vi "program seq..vi"(6 "IOList":T3, 7 "Cluster data":T6, 8 "DO":T4, 11 "Filepath":path=path "E:/My Project/2018-2019/Under development/Minda Ind. Switch -ID 144-145/Project/data/trail pro -12.txt") -> (0 "Error Out":errorcluster)   [LabVIEW 2015]
uses:
  Control PB/Active.ctl
  Control PB/deactive.ctl
  Control PB/output control.ctl
  Control PB/input control.ctl
  Control PB/timer.ctl
  Control PB/Remove list.ctl
  Control Button/Exit.ctl
  Control PB/Add_s.ctl
  Control PB/Delete_.ctl
  Control Button/Save.ctl
  Control PB/motor.ctl
  Data Acquisition/PCI-USB-DAQ/Digital out put.ctl
  Control PB/Camera.ctl
  Control PB/Barcode.ctl
  Galobal variable_TI.vi
panel:
  in  "Barcode 2":T1
  out "Step List 4":string[](array[string])
  out "Step List 3":string[](array[string])
  in  "Barcode":T1
  in  "Camera":T2
  out "x <= y?":bool
  out "Cancel":bool
  out "Step List 2":string[](array[string])
  out "Pokayoka Result":cluster{"Sensor Name":string, "Boolean":bool}[](array[cluster])
  in  "Feed Back Channel":i32[](listbox)=[0]
  out "Input":bool[](array[boolean])
  out "Feature List (Out) 2":T5(array[cluster])
  out "error out 2":errorcluster
  in  "Control":bool
  out "Station No":string
  out "Model Name":string
  out "Machine Name":string
  in  "Motor":T7
  in  "Feature List":i32(listbox) caption="Steps List"
  in  "Deletefeature list":T8
  in  "Add feature list":T9
  in  "Deactive":T10
  in  "Active":T11
  in  "Program step":i32(listbox)
  in  "Remove Step":T12
  in  "Wait Time":u32=100 caption="Timer(ms)" max=600000 step=1
  in  "Timer":T13
  in  "Save":T14
  in  "stop":T15
  in  "op Add":T16
  in  "Input Add":T17
  out "Step List":string[](array[string])
  out "output cluster":T18
  in  "Analog":bool
  in  "Analog Input":i32[](listbox)=[0]
  in  "Control Channel":i32[](listbox)=[7]
  in  "Steps":T19(array[cluster])
  in  "Program mode":string="Data"
  out "error out":errorcluster
  out "Feature List (Out)":T20(array[cluster])
  # "Program Sequence Window"
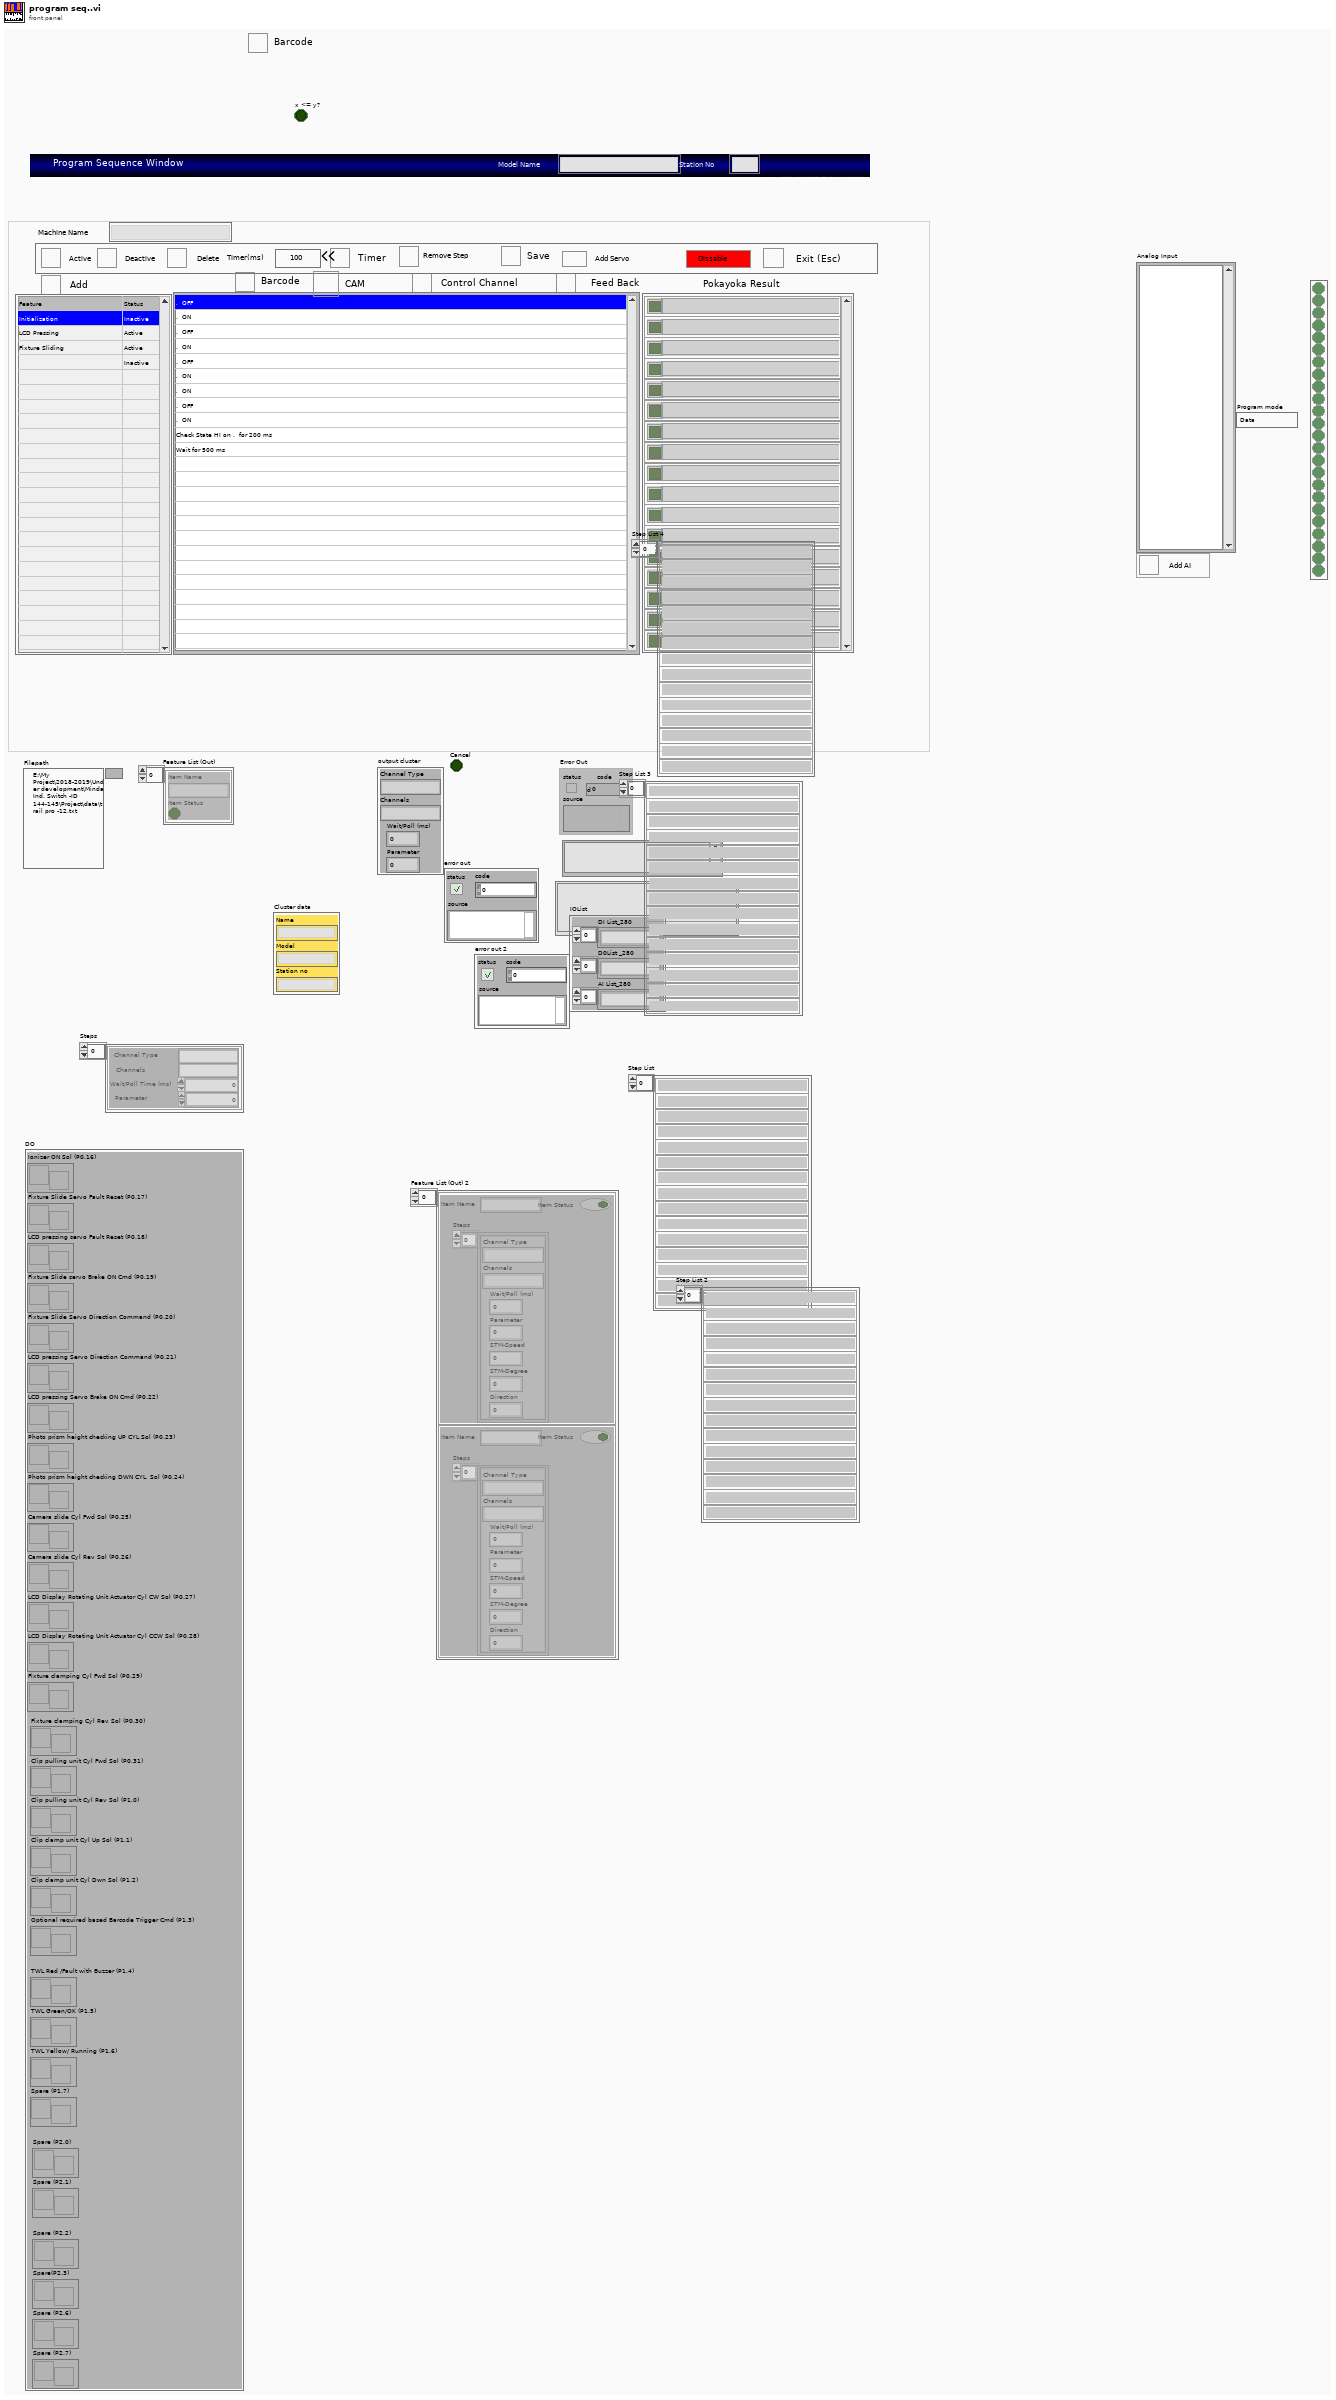
[diagram p1: front panel]
types:
  T1 = typedef "Barcode.ctl" = bool
  T2 = typedef "Camera.ctl" = bool
  T3 = cluster{"DI List_280":string[], "D0List _280":string[], "AI List_280":string[]}
  T4 = typedef "Digital out put.ctl" = cluster{"Ionizer ON Sol (P0.16)":refnum<notifier>, "Fixture Slide Servo Fault Reset (P0.17)":refnum<notifier>, "LCD pressing servo Fault Reset (P0.18)":refnum<notifier>, "Fixture Slide servo Brake ON Cmd (P0.19)":refnum<notifier>, "Fixture Slide Servo Direction Command (P0.20)":refnum<notifier>, "LCD pressing Servo Direction Command (P0.21)":refnum<notifier>, "LCD pressing Servo Brake ON Cmd (P0.22)":refnum<notifier>, "Photo prism height checking UP CYL Sol (P0.23)":refnum<notifier>, "Photo prism height checking DWN CYL  Sol (P0.24)":refnum<notifier>, "Camera slide Cyl Fwd Sol (P0.25)":refnum<notifier>, "Camera slide Cyl Rev Sol (P0.26)":refnum<notifier>, "LCD Display Rotating Unit Actuator Cyl CW Sol (P0.27)":refnum<notifier>, "LCD Display Rotating Unit Actuator Cyl CCW Sol (P0.28)":refnum<notifier>, "Fixture clamping Cyl Fwd Sol (P0.29)":refnum<notifier>, "Fixture clamping Cyl Rev Sol (P0.30)":refnum<notifier>, "Clip pulling unit Cyl Fwd Sol (P0.31)":refnum<notifier>, "Clip pulling unit Cyl Rev Sol (P1.0)":refnum<notifier>, "Clip clamp unit Cyl Up Sol (P1.1)":refnum<notifier>, "Clip clamp unit Cyl Dwn Sol (P1.2)":refnum<notifier>, "Optional required based Barcode Trigger Cmd (P1.3)":refnum<notifier>, "TWL Red /Fault with Buzzer (P1.4)":refnum<notifier>, "TWL Green/OK (P1.5)":refnum<notifier>, "TWL Yellow/ Running (P1.6)":refnum<notifier>, "Spare (P1.7)":refnum<notifier>, "Spare (P2.0)":refnum<notifier>, "Spare (P2.1)":refnum<notifier>, "Spare (P2.2)":refnum<notifier>, "Spare(P2.3)":refnum<notifier>, "Spare (P2.6)":refnum<notifier>, "Spare (P2.7) ":refnum<notifier>}
  T5 = cluster{"Item Name":string, "Item Status":bool, "Steps":cluster{"Channel Type":string, "Channels":string, "Wait/Poll (ms)":u32, "Parameter":u8, "STM-Speed":i32, "STM-Degree":u32, "Direction":u8}[]}[]
  T6 = cluster{"Name":string, "Model":string, "Station no":string}
  T7 = typedef "motor.ctl" = bool
  T8 = typedef "Delete_.ctl" = bool
  T9 = typedef "Add_s.ctl" = bool
  T10 = typedef "deactive.ctl" = bool
  T11 = typedef "Active.ctl" = bool
  T12 = typedef "Remove list.ctl" = bool
  T13 = typedef "timer.ctl" = bool
  T14 = typedef "Save.ctl" = bool
  T15 = typedef "Exit.ctl" = bool
  T16 = typedef "output control.ctl" = bool
  T17 = typedef "input control.ctl" = bool
  T18 = cluster{"Channel Type":string, "Channels":string, "Wait/Poll (ms)":u32, "Parameter":u8}
  T19 = cluster{"Channel Type":string, "Channels":string, "Wait/Poll Time (ms)":u32, "Parameter":u8}[]
  T20 = cluster{"Item Name":string, "Item Status":bool}[]
  T21 = cluster{"Channel Type":string, "Channels":string, "Wait/Poll (ms)":u32, "Parameter":u8, "STM-Speed":i32, "STM-Degree":i32, "Direction":u8}
  T22 = cluster{"Item Name":string, "Item Status":bool, "Steps":cluster{"Channel Type":string, "Channels":string, "Wait/Poll (ms)":u32, "Parameter":u8, "STM-Speed":i32, "STM-Degree":u32, "Direction":u8}[]}
  T23 = cluster{"Channel Type":string, "Channels":string, "Wait/Poll (ms)":u32, "Parameter":u8, "STM-Speed":i32, "STM-Degree":u32, "Direction":u8}[]
  T24 = cluster{"Item Name":string, "Active":T11, "Steps":cluster{"Channel Type":string, "Channels":string, "Wait/Poll (ms)":u32, "Parameter":u8, "STM-Speed":i32, "STM-Degree":u32, "Direction":u8}[]}
  T25 = cluster{"Channel Type":string, "Channels":string, "Wait/Poll (ms)":u32, "Parameter":u8, "STM-Speed":i32, "STM-Degree":i32, "Direction":u8}[]
  T26 = cluster{"Feature name ":string, bool, cluster{"Channel Type":string, "Channels":string, "Wait/Poll (ms)":u32, "Parameter":u8, "STM-Speed":i32, "STM-Degree":i32, "Direction":u8}[]}
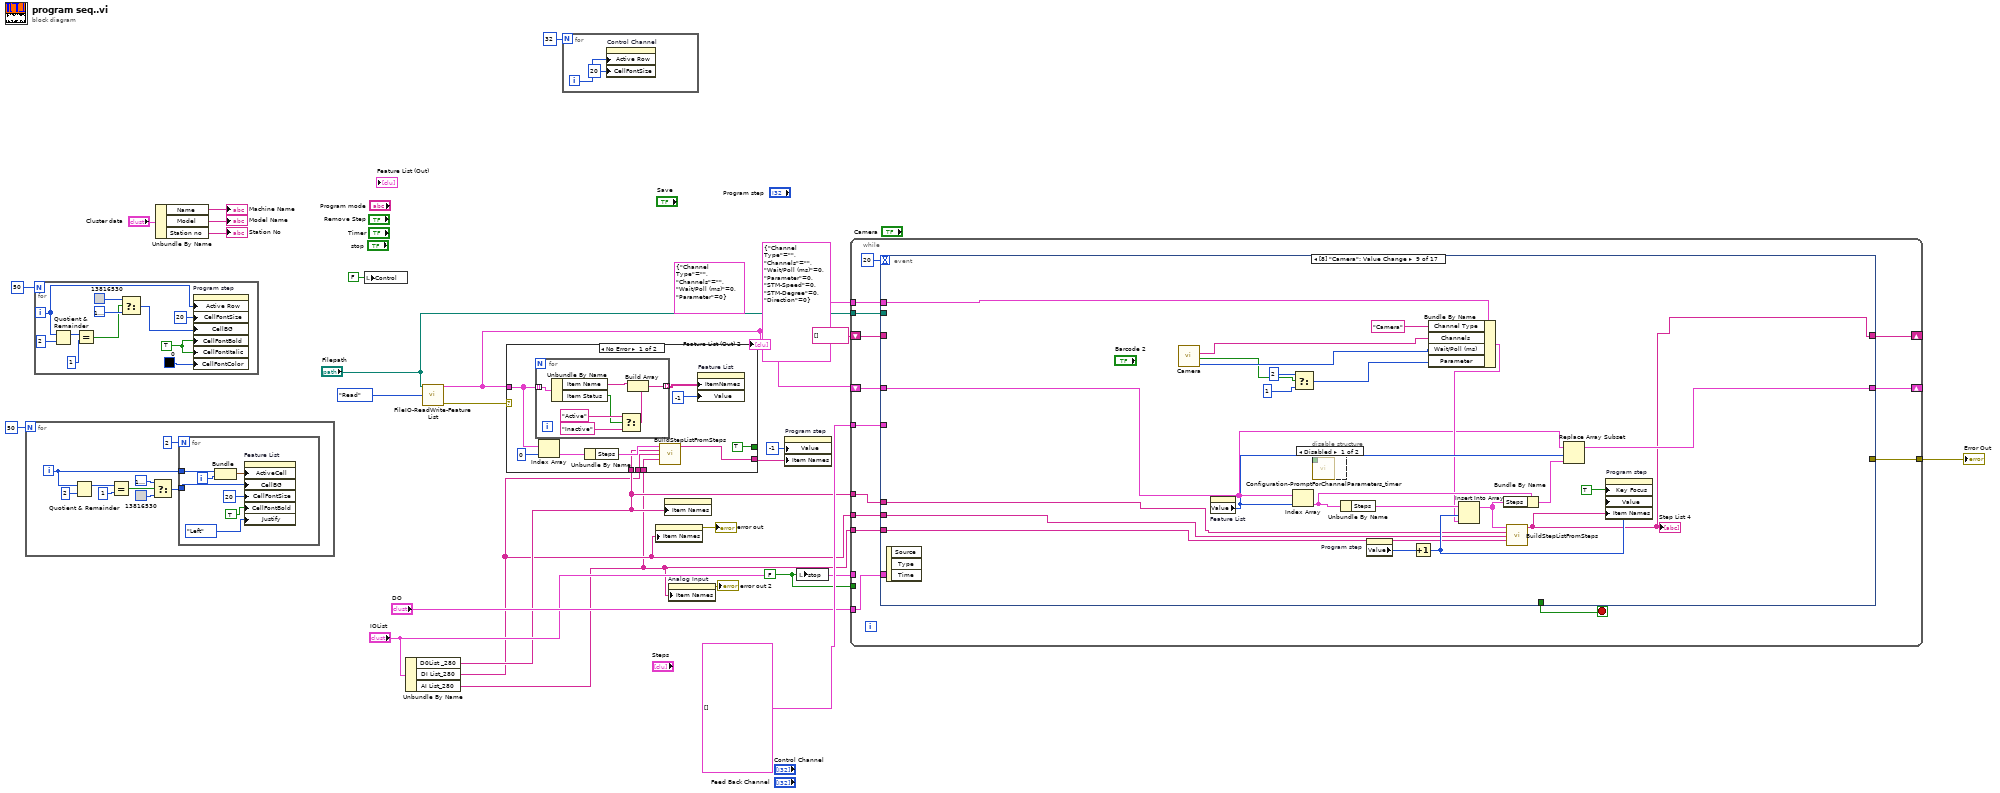
[diagram p0: block diagram]
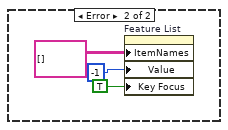
[diagram p2: hidden frame]
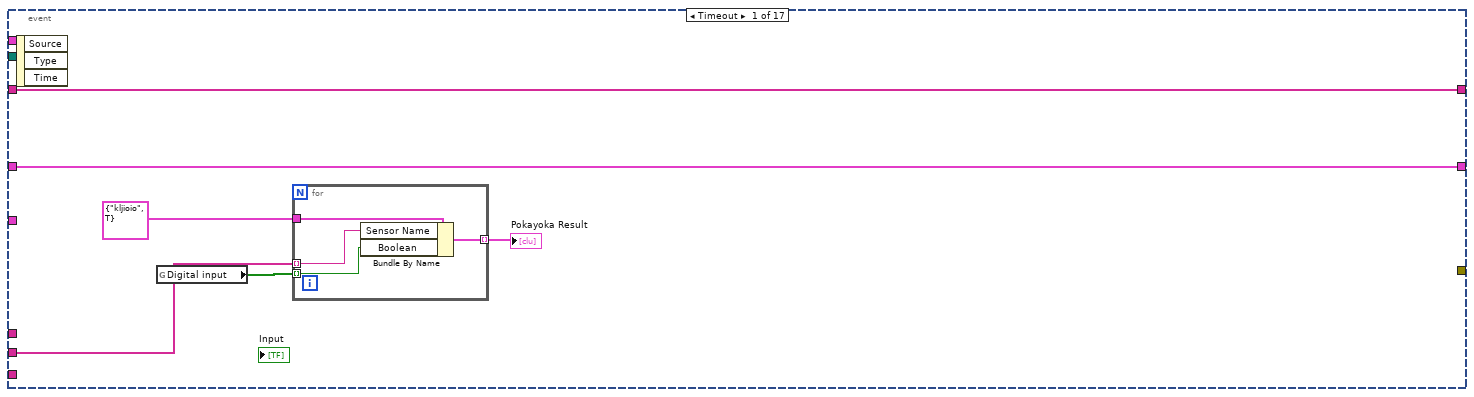
[diagram p3: hidden frame]
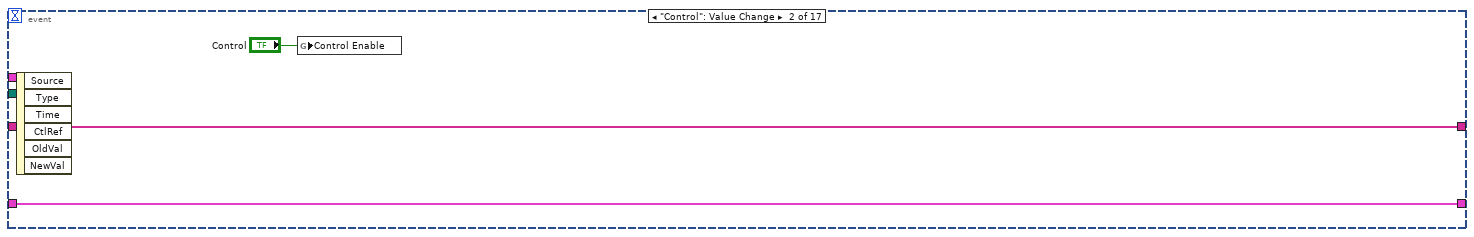
[diagram p4: hidden frame]
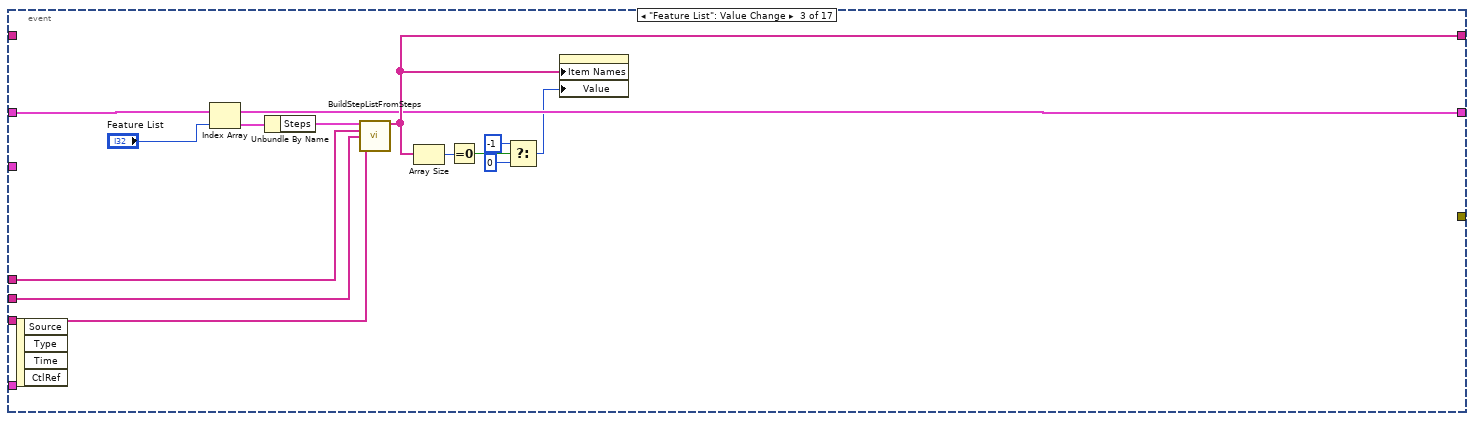
[diagram p5: hidden frame]
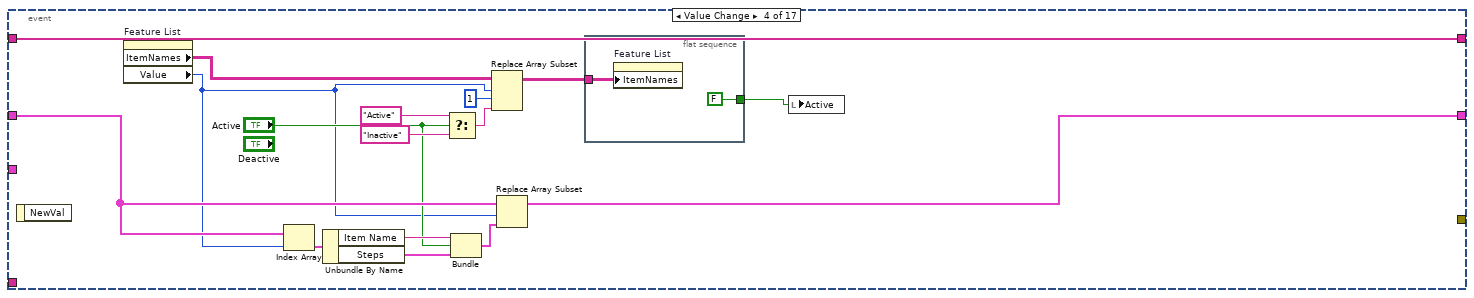
[diagram p6: hidden frame]
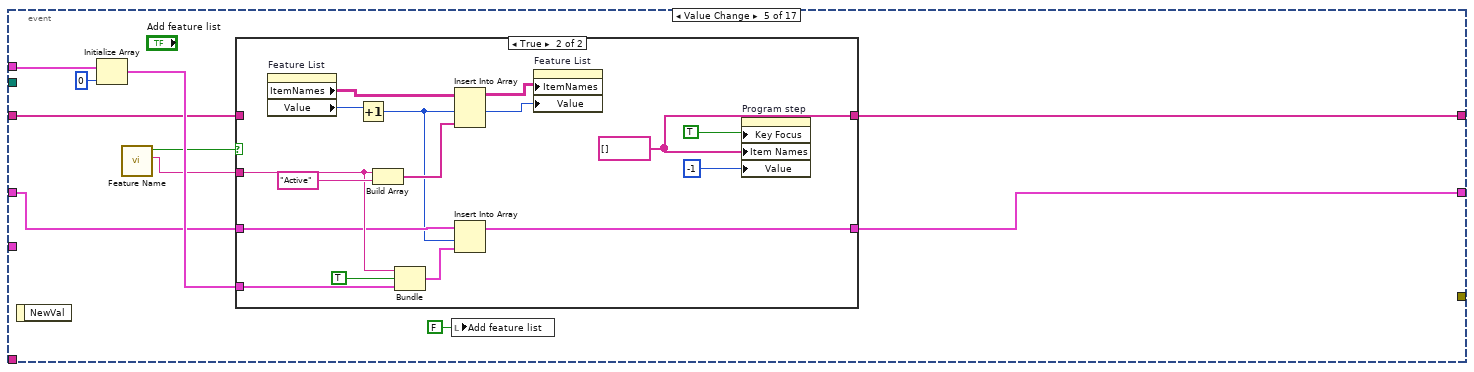
[diagram p7: hidden frame]
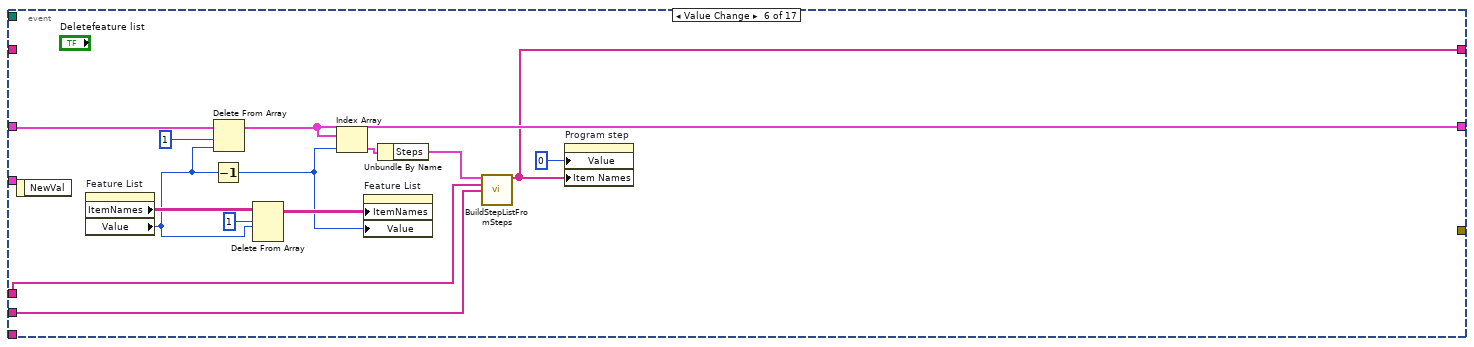
[diagram p9: hidden frame]
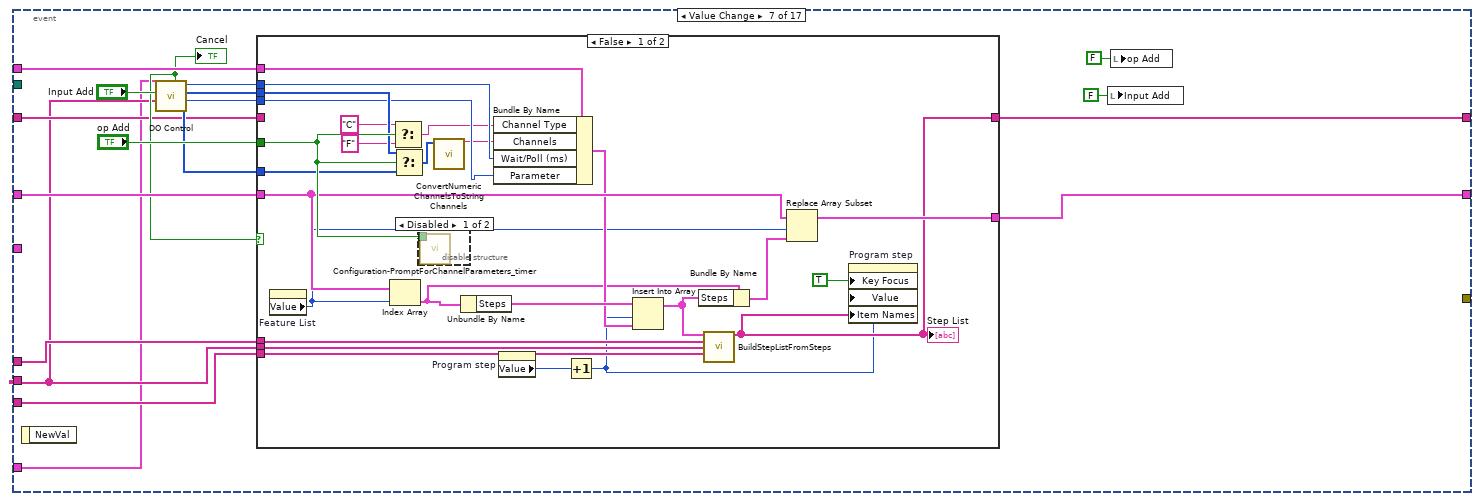
[diagram p10: hidden frame]
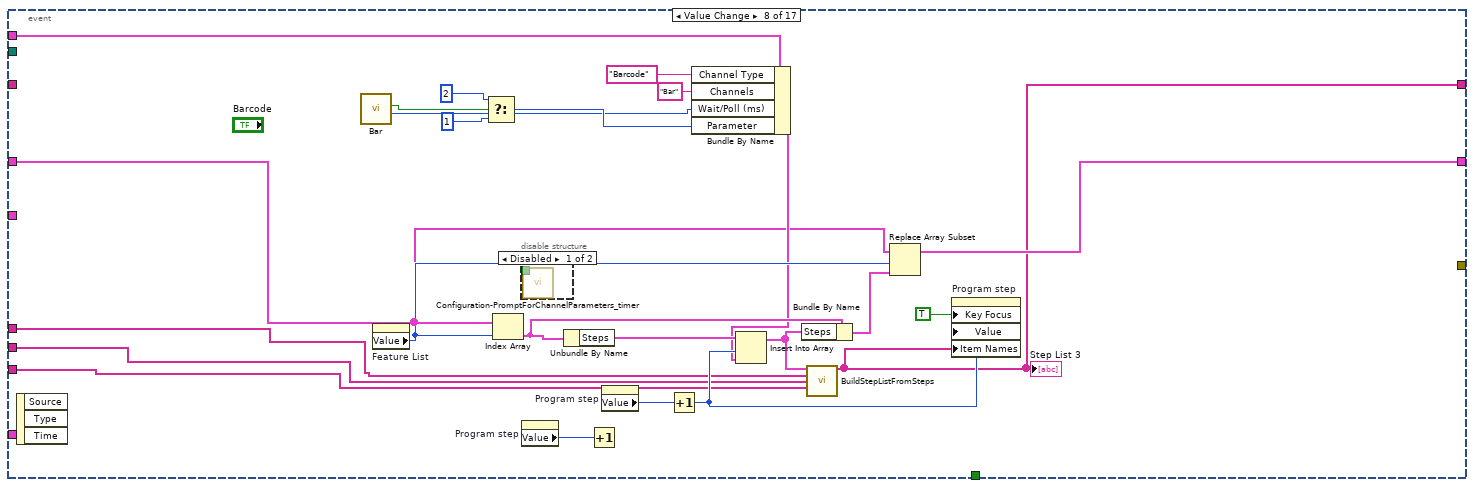
[diagram p13: hidden frame]
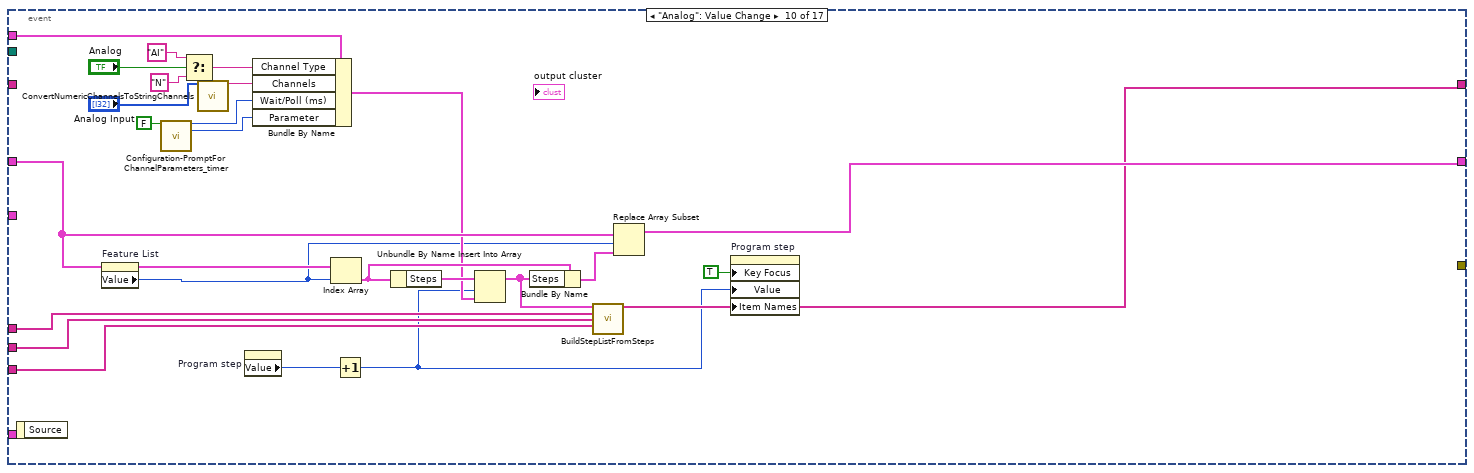
[diagram p16: hidden frame]
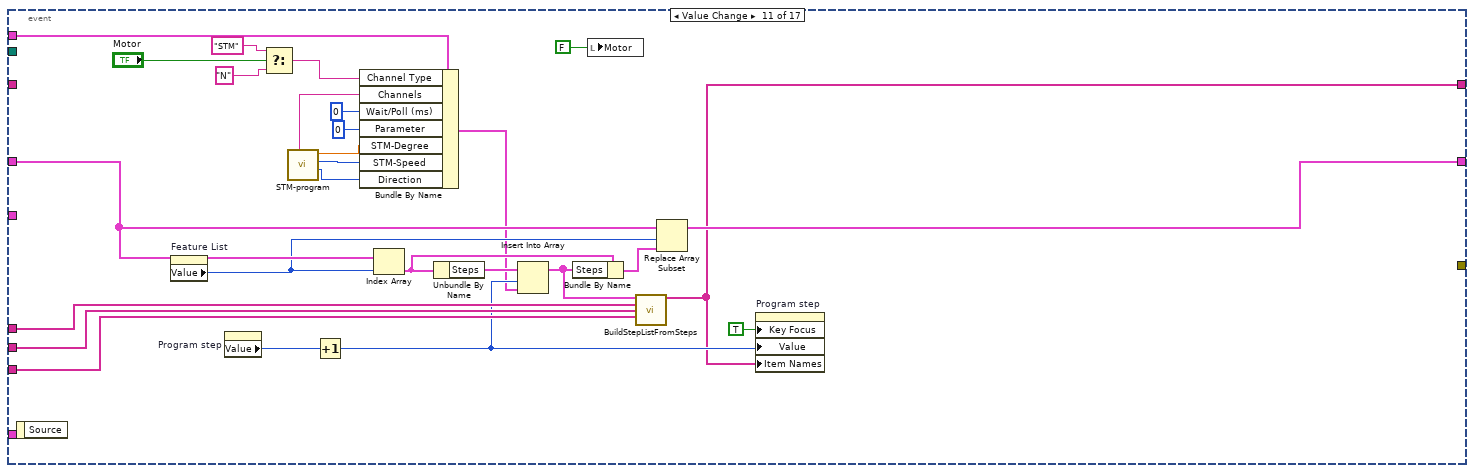
[diagram p17: hidden frame]
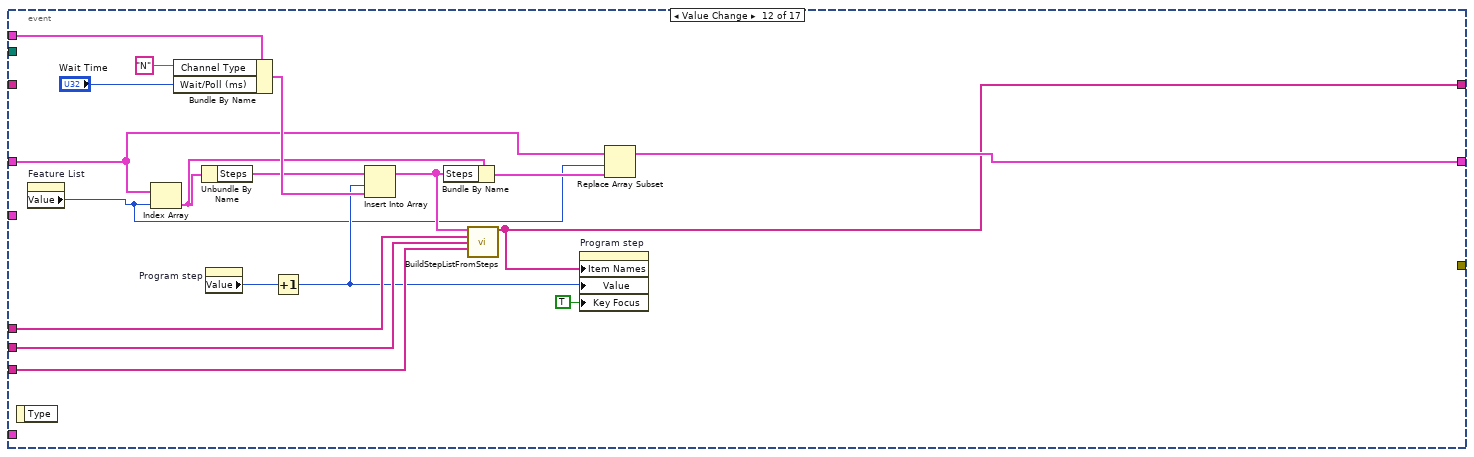
[diagram p18: hidden frame]
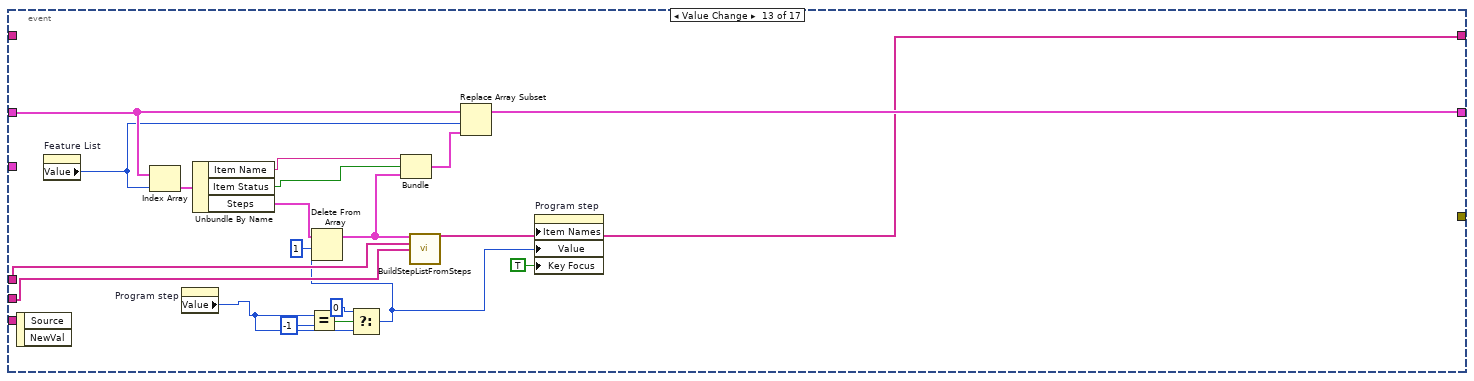
[diagram p19: hidden frame]
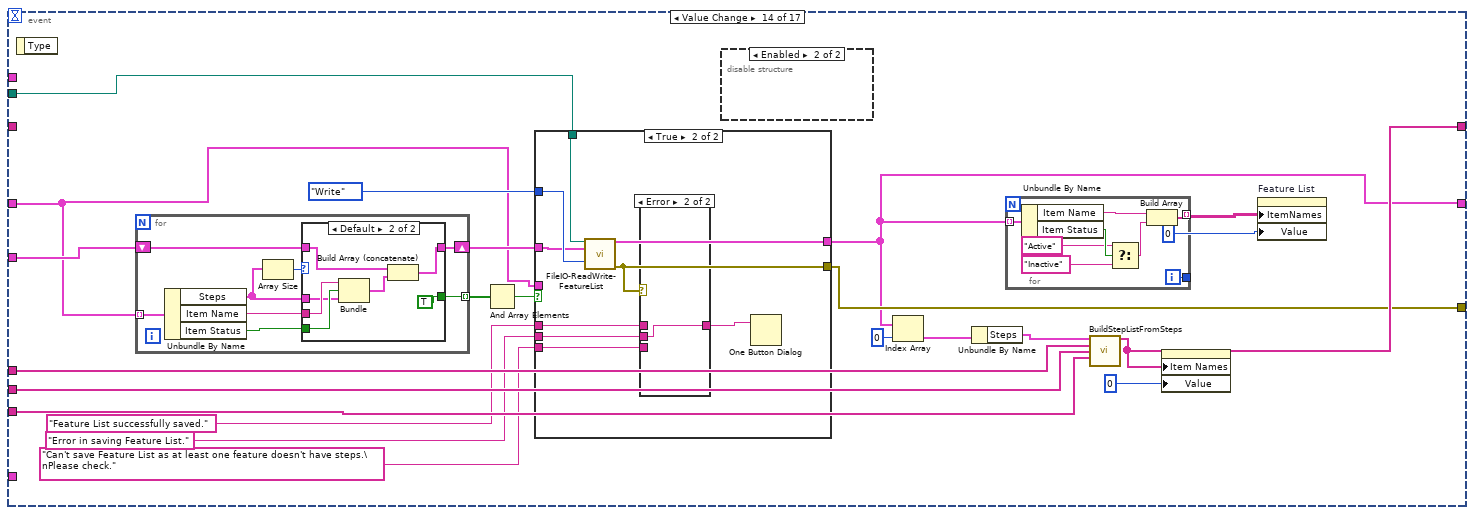
[diagram p20: hidden frame]
diagram:
  w9 = FALSE ("stop")
  (unwired) T18 {"Channel Type"="", "Channels"="", "Wait/Poll (ms)"=0, "Parameter"=0} ("Step")
  n1 = for {
    N: 50 -> [_]
    i -> [w34]
    n2 = Quotient & Remainder(x=w34, y=2) -> (x-y*floor(x/y)=w32:i32)  [unwired: 1 out]
    n3 = Equal?(x=w32, y=1) -> (x = y?=w30:bool)
    n4 = Select(t=u32 16777225 ("Color Box"), s=w30, f=u32 13816530 ("Color Box")) -> (s? t:f=w27:u32)
    n5 = for {
      N: 2 -> [_]
      tunnel: w34 -> [w42]
      tunnel: w27 -> [w39]
      i -> [w41]
      n6 = Bundle(w42, w41) -> (w40:cluster{i32, i32})  [unwired: 1 in]
      n7 = property on="Feature List" class="MCListbox (strict)"("ActiveCell"=w40, "CellBG"=w39, "CellFontSize"=u32 20 ("Active Cell:Cell Font:Size"), "CellFontBold"=TRUE ("Active Cell:Cell Font:Bold"), "Justify"=enum16{"Left", "Center", "Right"}."Left" ("Active Cell:Cell Justification")) -> ()  [unwired: 2 in, 2 out]
    }
  }
  n8 = for {
    N: 50 -> [_]
    i -> [w47]
    w44 = TRUE
    n9 = Quotient & Remainder(x=w47, y=2) -> (x-y*floor(x/y)=w50:i32)  [unwired: 1 out]
    n10 = Equal?(x=w50, y=1) -> (x = y?=w48:bool)
    n11 = Select(t=u32 13816530 ("Color Box"), s=w48, f=u32 16777226 ("Color Box")) -> (s? t:f=w45:u32)
    n12 = property on="Program step" class="LstBox (strict)"("Active Row"=w47, "CellFontSize"=u32 20 ("Active Row:Cell Font:Size"), "CellBG"=w45, "CellFontBold"=w44, "CellFontItalic"=w44, "CellFontColor"=u32 0 ("Color Box")) -> ()  [unwired: 2 in, 2 out]
  }
  n13 = Unbundle By Name("Cluster data") -> ("Name"=→"Machine Name":string, "Model"=→"Model Name":string, "Station no"=→"Station No":string)
  n14 = local write "Control"(FALSE ("Control")) -> ()
  n15 = Unbundle By Name("IOList") -> ("D0List _280"=w4:string[], "DI List_280"=w3:string[], "AI List_280"=w2:string[])
  n16 = call "FileIO-ReadWrite-FeatureList.vi"("Filepath"="Filepath", "Read/Write"=enum16{"Read", "Write"}."Read") -> ("Feature List (Out)"=w17:T5, "Error Out"=w21:errorcluster)  [unwired: 12 in]
  "Feature List (Out) 2" <- w17
  n17 = case shown="No Error" w21 {
    tunnel: w17 -> [w64 _]
    tunnel: w4 -> [w60 _]
    tunnel: w3 -> [w59 _]
    tunnel: w2 -> [w58 _]
    tunnel: [w57 _] -> w20
    tunnel: [TRUE ("Key Focus") _] -> _
    frame No Error {
      n18 = for {
        tunnel: w64 -> [w71] mode=indexing
        tunnel: [w65] -> w55 mode=indexing
        n19 = Unbundle By Name(w71) -> ("Item Name"=w67:string, "Item Status"=w68:bool)
        n20 = Select(t="Active", s=w68, f="Inactive") -> (s? t:f=w66:string)
        n21 = Build Array(w67, w66) -> (w65:string[])
      }
      n22 = Index Array(array=w64, index=0) -> (element=w62:T22)
      n23 = Unbundle By Name(w62) -> ("Steps"=w61:T23)
      n24 = call "BuildStepListFromSteps.vi"("Steps"=w61, "Control Channels"=w60, "Feedback Channels"=w59, "AI"=w58) -> ("Step List"=w57:string[])  [unwired: 11 in]
      n25 = property on="Feature List" class="MCListbox (strict)"("ItemNames"=w55, "Value"=-1 ("Feautre list")) -> ()  [unwired: 2 in, 2 out]
    }
    frame Error {
      n26 = property on="Feature List" class="MCListbox (strict)"("ItemNames"=string[][] [] ("Item Names"), "Value"=-1 ("Feautre list"), "Key Focus"=TRUE) -> ()  [unwired: 2 in, 2 out]
    }
  }
  n27 = for {
    N: 32 -> [_]
    i -> [w76]
    n28 = property on="Control Channel" class="LstBox (strict)"("Active Row"=w76, "CellFontSize"=u32 20 ("Active Row:Cell Font:Size")) -> ()  [unwired: 2 in, 2 out]
  }
  n29 = property on="Feed Back Channel" class="LstBox (strict)"("Item Names"=w3) -> (error out=→"error out":errorcluster)  [unwired: 2 in, 1 out]
  n30 = property on="Control Channel" class="LstBox (strict)"("Item Names"=w4) -> ()  [unwired: 2 in, 2 out]
  n31 = property on="Analog Input" class="LstBox (strict)"("Item Names"=w2) -> (error out=→"error out 2":errorcluster)  [unwired: 2 in, 1 out]
  n32 = property on="Program step" class="LstBox (strict)"("Value"=-1 ("Step feautre list"), "Item Names"=w20) -> ()  [unwired: 2 in, 2 out]
  n33 = local write "stop"(w9) -> ()
  n34 = while {
    shift-right: [w88] -> _
    shift-left: w17 -> [w79]
    tunnel: T21 {"Channel Type"="", "Channels"="", "Wait/Poll (ms)"=0, "Parameter"=0, "STM-Speed"=0, "STM-Degree"=0, "Direction"=0} ("Step") -> [w89]
    shift-right: [w87] -> _
    shift-left: string[] [] ("Step List") -> [w86]
    tunnel: w4 -> [w85]
    tunnel: w3 -> [w84]
    tunnel: [w83] -> w24
    tunnel: w2 -> [w82]
    tunnel: T5 [] ("Feature List (Out) 2") -> [w81]
    tunnel: "Filepath" -> [w80]
    tunnel: w9 -> [_]
    tunnel: "DO" -> [w78]
    tunnel: "IOList" -> [_]
    stop <- w90 stop-if-true
    n35 = event shown="[8] \"Camera\": Value Change" {
      selector: _ -> [_ _ _ _ _ _ _ _ _ _ _ _ _ _ _ _ _]
      dyn-events: _ -> [_ _ _ _ _ _ _ _ _ _ _ _ _ _ _ _ _]
      timeout: 20 -> [_ _ _ _ _ _ _ _ _ _ _ _ _ _ _ _ _]
      tunnel: [_ _ _ _ _ _ _ _ _ _ _ _ _ _ TRUE ("stop") _ TRUE ("Discard?")] -> w90
      tunnel: w79 -> [w96 w102 w107 w124 w141 w173 w190 w226 w253 w281 w311 w332 w354 w363 w423 w445 w522]
      tunnel: w89 -> [_ _ _ _ w144 _ w193 w246 w257 w288 w316 w341 _ _ _ w446 _]
      tunnel: [w96 w102 w107 w122 w140 w172 w191 w225 w252 w276 w303 w331 w353 w365 w423 w441 w522] -> w88
      tunnel: [w95 w103 w110 w121 w137 w167 w188 w224 w251 w275 w302 w328 w348 w380 w422 w440 w523] -> w87
      tunnel: w86 -> [w95 w103 _ w121 w136 _ w178 _ _ _ _ _ _ _ w422 w439 w523]
      tunnel: w85 -> [_ _ w109 _ _ w169 w189 w227 w254 w278 w308 w330 w350 w382 _ w442 _]
      tunnel: w84 -> [w94 _ w108 _ _ w168 w177 w228 w255 w279 w307 w329 w349 w381 _ w443 _]
      tunnel: [_ _ _ _ _ _ _ _ _ _ _ _ _ w373 _ _ _] -> w83
      tunnel: w82 -> [_ _ w106 _ _ _ w187 w229 w256 w280 w306 w327 _ w374 _ w444 _]
      tunnel: w81 -> [_ _ _ _ _ _ _ _ _ _ _ _ _ w379 _ _ _]
      tunnel: w80 -> [_ _ _ _ _ _ _ _ _ _ _ _ _ w364 _ _ _]
      tunnel: w78 -> [_ _ _ _ _ _ w176 _ _ _ _ _ _ _ _ _ _]
      event Timeout {
        n36 = event-data() -> ()  [unwired: 1 in, 3 out]
        n37 = global read "Galobal variable_TI.vi" "Digital input"() -> (w91:bool[])
        n38 = for {
          tunnel: w94 -> [w99] mode=indexing
          tunnel: cluster{"Sensor Name":string, "Boolean":bool} {"Sensor Name"="kljioio", "Boolean"=TRUE} ("Cluster") -> [w100]
          tunnel: [w98] -> w92 mode=indexing
          tunnel: w91 -> [w97] mode=indexing
          n39 = Bundle By Name(cluster=w100, "Sensor Name"=w99, "Boolean"=w97) -> (w98:cluster{"Sensor Name":string, "Boolean":bool})
        }
        "Pokayoka Result" <- w92
      }
      event "Control": Value Change {
        n40 = event-data() -> ()  [unwired: 1 in, 6 out]
        n41 = global write "Galobal variable_TI.vi" "Control Enable"("Control") -> ()
      }
      event "Feature List": Value Change {
        n42 = event-data() -> ()  [unwired: 1 in, 4 out]
        n43 = Index Array(array=w107, index="Feature List") -> (element=w116:T22)
        n44 = Unbundle By Name(w116) -> ("Steps"=w115:T23)
        n45 = call "BuildStepListFromSteps.vi"("Steps"=w115, "Control Channels"=w109, "Feedback Channels"=w108, "AI"=w106) -> ("Step List"=w110:string[])  [unwired: 11 in]
        n46 = Array Size(array=w110) -> (size(s)=w112:i32)
        n47 = Equal To 0?(x=w112) -> (x = 0?=w114:bool)
        n48 = Select(t=-1 ("Step List"), s=w114, f=0 ("Step List")) -> (s? t:f=w105:i32)
        n49 = property on="Program step" class="LstBox (strict)"("Item Names"=w110, "Value"=w105) -> ()  [unwired: 2 in, 2 out]
      }
      event Value Change {
        n50 = event-data() -> ()  [unwired: 1 in, 1 out]
        n51 = property on="Feature List" class="MCListbox (strict)"() -> ("ItemNames"=w120:string[][], "Value"=w118:i32)  [unwired: 2 in, 2 out]
        n52 = Index Array(array=w124, index=w118) -> (element=w130:T22)
        n53 = Unbundle By Name(w130) -> ("Item Name"=w131:string, "Steps"=w132:T23)
        n54 = Select(t="Active", s="Active", f="Inactive" ("element")) -> (s? t:f=w127:string)
        n55 = Bundle("Item Name"=w131, "Active"="Active", "Steps"=w132) -> (w129:T24)  [unwired: 1 in]
        n56 = Replace Array Subset(array=w120, new element=w127, index (row)=w118, index (col)=1 ("disabled index (col)")) -> (w119:string[][])
        n57 = Replace Array Subset(array=w124, new element=w129, index=w118) -> (w122:T5)
        n58 = flat-sequence {
          tunnel: w119 -> [w134]
          tunnel: [T11 FALSE ("Active")] -> w117
          frame #0 {
            n59 = property on="Feature List" class="MCListbox (strict)"("ItemNames"=w134) -> ()  [unwired: 2 in, 2 out]
          }
        }
        n60 = local write "Active"(w117) -> ()
      }
      event Value Change {
        n61 = event-data() -> ()  [unwired: 1 in, 1 out]
        n62 = Initialize Array(w144, 0 ("dimension size")) -> (w142:T25)
        n63 = call "Feature Name.vi"() -> ("Feature name"=w138:string, "Out"=w139:bool)  [unwired: 10 in]
        n64 = case shown="True" w139 {
          tunnel: w142 -> [_ w160]
          tunnel: w141 -> [w146 w155]
          tunnel: [w146 w157] -> w140
          tunnel: w138 -> [_ w156]
          tunnel: [w145 w153] -> w137
          tunnel: w136 -> [w145 _]
          frame False {
          }
          frame True {
            w153 = string[] [] ("Item Names")
            n65 = property on="Feature List" class="MCListbox (strict)"() -> ("ItemNames"=w150:string[][], "Value"=w147:i32)  [unwired: 2 in, 2 out]
            n66 = Increment(x=w147) -> (x+1=w148:i32)
            n67 = Build Array(w156, "Active") -> (w151:string[])
            n68 = Bundle("Feature name"=w156, TRUE, w160) -> (w158:T26)  [unwired: 1 in]
            n69 = Insert Into Array(array=w150, index (row)=w148, new element=w151) -> (w149:string[][])  [unwired: 1 in]
            n70 = Insert Into Array(array=w155, index=w148, new element=w158) -> (w157:T5)
            n71 = property on="Feature List" class="MCListbox (strict)"("ItemNames"=w149, "Value"=w148) -> ()  [unwired: 2 in, 2 out]
            n72 = property on="Program step" class="LstBox (strict)"("Key Focus"=TRUE, "Item Names"=w153, "Value"=-1 ("Step feautre list")) -> ()  [unwired: 2 in, 2 out]
          }
        }
        n73 = local write "Add feature list"(FALSE ("Add feature list")) -> ()
      }
      event Value Change {
        n74 = event-data() -> ()  [unwired: 1 in, 1 out]
        n75 = property on="Feature List" class="MCListbox (strict)"() -> ("ItemNames"=w165:string[][], "Value"=w164:i32)  [unwired: 2 in, 2 out]
        n76 = Decrement(x=w164) -> (x-1=w162:i32)
        n77 = Delete From Array(array=w173, length=1, index=w164) -> (array with subset deleted=w172:T5)  [unwired: 1 out]
        n78 = Delete From Array(array=w165, length=1, index (row)=w164) -> (array with subset deleted=w163:string[][])  [unwired: 1 in, 1 out]
        n79 = Index Array(array=w172, index=w162) -> (element=w171:T22)
        n80 = property on="Feature List" class="MCListbox (strict)"("ItemNames"=w163, "Value"=w162) -> ()  [unwired: 2 in, 2 out]
        n81 = Unbundle By Name(w171) -> ("Steps"=w170:T23)
        n82 = call "BuildStepListFromSteps.vi"("Steps"=w170, "Control Channels"=w169, "Feedback Channels"=w168) -> ("Step List"=w167:string[])  [unwired: 12 in]
        n83 = property on="Program step" class="LstBox (strict)"("Value"=0 ("Step feautre list"), "Item Names"=w167) -> ()  [unwired: 2 in, 2 out]
      }
      event Value Change {
        n84 = event-data() -> ()  [unwired: 1 in, 1 out]
        n85 = call "DO Control.vi"("DI List_280"=w177, "s"="Input Add", "DO"=w176) -> ("Feedback"=w182:i32[], "Parameter (Out)"=w184:u8, "Control Channel 2"=w186:i32[], "Poll Time (Out)"=w185:u32, "Cancel"=w179:bool)  [unwired: 3 in, 1 out]
        "Cancel" <- w179
        n86 = case shown="False" w179 {
          tunnel: w193 -> [w219 _]
          tunnel: "op Add" -> [w218 _]
          tunnel: [w217 w222] -> w191
          tunnel: w190 -> [w216 w222]
          tunnel: w189 -> [w215 _]
          tunnel: w177 -> [w214 _]
          tunnel: [w213 w221] -> w188
          tunnel: w187 -> [w212 _]
          tunnel: w186 -> [w211 _]
          tunnel: w185 -> [w210 _]
          tunnel: w184 -> [w209 _]
          tunnel: w182 -> [w208 _]
          tunnel: w178 -> [_ w221]
          frame False {
            n87 = property on="Feature List" class="MCListbox (strict)"() -> ("Value"=w194:i32)  [unwired: 2 in, 2 out]
            n88 = Index Array(array=w216, index=w194) -> (element=w200:T22)
            n89 = Select(t="C", s=w218, f="F") -> (s? t:f=w205:string)
            n90 = Select(t=w211, s=w218, f=w208) -> (s? t:f=w204:i32[])
            n91 = disable-structure shown="Disabled" {
              disable-tunnel: w218 -> [w220 _]
              frame Disabled {
                n92 = call "Configuration-PromptForChannelParameters_timer.vi"("Control/Feedback\n(Default: False = Feedback)"=w220) -> ()  [unwired: 13 in, 2 out]
              }
              frame Enabled {
              }
            }
            n93 = call "ConvertNumericChannelsToStringChannels.vi"("Channels (In)"=w204) -> ("Channels (A:B:C:D...) (Out)"=w203:string)  [unwired: 14 in]
            n94 = Unbundle By Name(w200) -> ("Steps"=w202:T23)
            n95 = Bundle By Name(cluster=w219, "Channel Type"=w205, "Channels"=w203, "Wait/Poll (ms)"=w210, "Parameter"=w209) -> (w201:T21)
            n96 = property on="Program step" class="LstBox (strict)"() -> ("Value"=w195:i32)  [unwired: 2 in, 2 out]
            n97 = Increment(x=w195) -> (x+1=w196:i32)
            n98 = Insert Into Array "Insert Into Array"(array=w202, index=w196, new element=w201) -> (w198:T23)
            n99 = Bundle By Name(cluster=w200, "Steps"=w198) -> (w199:T22)
            n100 = call "BuildStepListFromSteps.vi"("Steps"=w198, "Control Channels"=w215, "Feedback Channels"=w214, "AI"=w212) -> ("Step List"=w213:string[])  [unwired: 11 in]
            "Step List" <- w213
            n101 = Replace Array Subset(array=w216, new element=w199, index=w194) -> (w217:T5)
            n102 = property on="Program step" class="LstBox (strict)"("Key Focus"=TRUE, "Value"=w196, "Item Names"=w213) -> ()  [unwired: 2 in, 2 out]
          }
          frame True {
          }
        }
        n103 = local write "Input Add"(T17 FALSE ("Input Add")) -> ()
        n104 = local write "op Add"(T16 FALSE ("op Add")) -> ()
      }
      event Value Change {
        n105 = event-data() -> ()  [unwired: 1 in, 3 out]
        n106 = call "Bar.vi"() -> ("Time Out Value"=w223:u8, "Barcode Scane"=w243:bool)  [unwired: 9 in, 1 out]
        n107 = property on="Feature List" class="MCListbox (strict)"() -> ("Value"=w232:i32)  [unwired: 2 in, 2 out]
        n108 = Select(t=2, s=w243, f=1) -> (s? t:f=w240:i32)
        n109 = Index Array(array=w226, index=w232) -> (element=w238:T22)
        n110 = disable-structure shown="Disabled" {
          disable-tunnel: _ -> [w247 _]
          frame Disabled {
            n111 = call "Configuration-PromptForChannelParameters_timer.vi"("Control/Feedback\n(Default: False = Feedback)"=w247) -> ()  [unwired: 13 in, 2 out]
          }
          frame Enabled {
          }
        }
        n112 = property on="Program step" class="LstBox (strict)"() -> ("Value"=w231:i32)  [unwired: 2 in, 2 out]
        n113 = Unbundle By Name(w238) -> ("Steps"=w239:T23)
        n114 = Increment(x=w231) -> ()  [unwired: 1 out]
        n115 = property on="Program step" class="LstBox (strict)"() -> ("Value"=w233:i32)  [unwired: 2 in, 2 out]
        n116 = Increment(x=w233) -> (x+1=w234:i32)
        n117 = Bundle By Name(cluster=w246, "Channel Type"="Barcode", "Channels"="Bar", "Wait/Poll (ms)"=w223, "Parameter"=w240) -> (w230:T21)
        n118 = Insert Into Array "Insert Into Array"(array=w239, index=w234, new element=w230) -> (w236:T23)
        n119 = Bundle By Name(cluster=w238, "Steps"=w236) -> (w237:T22)
        n120 = call "BuildStepListFromSteps.vi"("Steps"=w236, "Control Channels"=w227, "Feedback Channels"=w228, "AI"=w229) -> ("Step List"=w224:string[])  [unwired: 11 in]
        "Step List 3" <- w224
        n121 = Replace Array Subset(array=w226, new element=w237, index=w232) -> (w225:T5)
        n122 = property on="Program step" class="LstBox (strict)"("Key Focus"=TRUE, "Value"=w234, "Item Names"=w224) -> ()  [unwired: 2 in, 2 out]
      }
      event Value Change {
        n123 = event-data() -> ()  [unwired: 1 in, 3 out]
        n124 = call "Camera.vi"() -> ("Time Out (ms) 2"=w249:u8, "Camera 2"=w248:bool, "Feature name"=w250:string)  [unwired: 8 in, 1 out]
        n125 = property on="Feature List" class="MCListbox (strict)"() -> ("Value"=w259:i32)  [unwired: 2 in, 2 out]
        n126 = Index Array(array=w253, index=w259) -> (element=w265:T22)
        n127 = Select(t=2, s=w248, f=1) -> (s? t:f=w267:i32)
        n128 = disable-structure shown="Disabled" {
          disable-tunnel: _ -> [w271 _]
          frame Disabled {
            n129 = call "Configuration-PromptForChannelParameters_timer.vi"("Control/Feedback\n(Default: False = Feedback)"=w271) -> ()  [unwired: 13 in, 2 out]
          }
          frame Enabled {
          }
        }
        n130 = Unbundle By Name(w265) -> ("Steps"=w266:T23)
        n131 = property on="Program step" class="LstBox (strict)"() -> ("Value"=w260:i32)  [unwired: 2 in, 2 out]
        n132 = Increment(x=w260) -> (x+1=w261:i32)
        n133 = Bundle By Name(cluster=w257, "Channel Type"="Camera", "Channels"=w250, "Wait/Poll (ms)"=w249, "Parameter"=w267) -> (w258:T21)
        n134 = Insert Into Array "Insert Into Array"(array=w266, index=w261, new element=w258) -> (w263:T23)
        n135 = Bundle By Name(cluster=w265, "Steps"=w263) -> (w264:T22)
        n136 = call "BuildStepListFromSteps.vi"("Steps"=w263, "Control Channels"=w254, "Feedback Channels"=w255, "AI"=w256) -> ("Step List"=w251:string[])  [unwired: 11 in]
        "Step List 4" <- w251
        n137 = Replace Array Subset(array=w253, new element=w264, index=w259) -> (w252:T5)
        n138 = property on="Program step" class="LstBox (strict)"("Key Focus"=TRUE, "Value"=w261, "Item Names"=w251) -> ()  [unwired: 2 in, 2 out]
      }
      event "Analog": Value Change {
        n139 = event-data() -> ()  [unwired: 1 in, 1 out]
        n140 = property on="Feature List" class="MCListbox (strict)"() -> ("Value"=w272:i32)  [unwired: 2 in, 2 out]
        n141 = call "Configuration-PromptForChannelParameters_timer.vi"("Control/Feedback\n(Default: False = Feedback)"=FALSE ("Control/Feedback\n(Default: False = Feedback)")) -> ("Poll Time (Out)"=w292:u32, "Parameter (Out)"=w291:u8)  [unwired: 13 in]
        n142 = Select(t="AI", s="Analog", f="N") -> (s? t:f=w294:string)
        n143 = call "ConvertNumericChannelsToStringChannels.vi"("Channels (In)"="Analog Input") -> ("Channels (A:B:C:D...) (Out)"=w293:string)  [unwired: 14 in]
        n144 = property on="Program step" class="LstBox (strict)"() -> ("Value"=w282:i32)  [unwired: 2 in, 2 out]
        n145 = Bundle By Name(cluster=w288, "Channel Type"=w294, "Channels"=w293, "Wait/Poll (ms)"=w292, "Parameter"=w291) -> (w277:T21)
        n146 = Index Array(array=w281, index=w272) -> (element=w286:T22)
        n147 = Increment(x=w282) -> (x+1=w273:i32)
        n148 = Unbundle By Name(w286) -> ("Steps"=w287:T23)
        n149 = Insert Into Array(array=w287, index=w273, new element=w277) -> (w284:T23)
        n150 = Bundle By Name(cluster=w286, "Steps"=w284) -> (w285:T22)
        n151 = call "BuildStepListFromSteps.vi"("Steps"=w284, "Control Channels"=w278, "Feedback Channels"=w279, "AI"=w280) -> ("Step List"=w275:string[])  [unwired: 11 in]
        n152 = Replace Array Subset(array=w281, new element=w285, index=w272) -> (w276:T5)
        n153 = property on="Program step" class="LstBox (strict)"("Key Focus"=TRUE, "Value"=w273, "Item Names"=w275) -> ()  [unwired: 2 in, 2 out]
      }
      event Value Change {
        n154 = event-data() -> ()  [unwired: 1 in, 1 out]
        n155 = property on="Feature List" class="MCListbox (strict)"() -> ("Value"=w310:i32)  [unwired: 2 in, 2 out]
        n156 = property on="Program step" class="LstBox (strict)"() -> ("Value"=w309:i32)  [unwired: 2 in, 2 out]
        n157 = Select(t="STM", s="Motor", f="N") -> (s? t:f=w321:string)
        n158 = call "STM-program.vi"() -> ("OutDir"=w320:i32, "Out Speed"=w318:i32, "Out Degree"=w319:dbl, "Channels (A:B:C:D...) (Out)"=w298:string)  [unwired: 7 in, 1 out]
        n159 = Increment(x=w309) -> (x+1=w304:i32)
        n160 = Bundle By Name(cluster=w316, "Channel Type"=w321, "Channels"=w298, "Wait/Poll (ms)"=u32 0, "Parameter"=u8 0, "STM-Degree"=w319, "STM-Speed"=w318, "Direction"=w320) -> (w301:T21)
        n161 = Index Array(array=w311, index=w310) -> (element=w314:T22)
        n162 = Unbundle By Name(w314) -> ("Steps"=w315:T23)
        n163 = Insert Into Array(array=w315, index=w304, new element=w301) -> (w312:T23)
        n164 = Bundle By Name(cluster=w314, "Steps"=w312) -> (w313:T22)
        n165 = local write "Motor"(FALSE ("Motor")) -> ()
        n166 = call "BuildStepListFromSteps.vi"("Steps"=w312, "Control Channels"=w308, "Feedback Channels"=w307, "AI"=w306) -> ("Step List"=w302:string[])  [unwired: 11 in]
        n167 = Replace Array Subset(array=w311, new element=w313, index=w310) -> (w303:T5)
        n168 = property on="Program step" class="LstBox (strict)"("Key Focus"=TRUE, "Value"=w304, "Item Names"=w302) -> ()  [unwired: 2 in, 2 out]
      }
      event Value Change {
        n169 = event-data() -> ()  [unwired: 1 in, 1 out]
        n170 = property on="Feature List" class="MCListbox (strict)"() -> ("Value"=w324:i32)  [unwired: 2 in, 2 out]
        n171 = Index Array(array=w332, index=w324) -> (element=w335:T22)
        n172 = Bundle By Name(cluster=w341, "Channel Type"="N", "Wait/Poll (ms)"="Wait Time") -> (w337:T21)
        n173 = Unbundle By Name(w335) -> ("Steps"=w336:T23)
        n174 = property on="Program step" class="LstBox (strict)"() -> ("Value"=w338:i32)  [unwired: 2 in, 2 out]
        n175 = Increment(x=w338) -> (x+1=w325:i32)
        n176 = Insert Into Array(array=w336, index=w325, new element=w337) -> (w333:T23)
        n177 = Bundle By Name(cluster=w335, "Steps"=w333) -> (w334:T22)
        n178 = call "BuildStepListFromSteps.vi"("Steps"=w333, "Control Channels"=w330, "Feedback Channels"=w329, "AI"=w327) -> ("Step List"=w328:string[])  [unwired: 11 in]
        n179 = property on="Program step" class="LstBox (strict)"("Item Names"=w328, "Value"=w325, "Key Focus"=TRUE) -> ()  [unwired: 2 in, 2 out]
        n180 = Replace Array Subset(array=w332, new element=w334, index=w324) -> (w331:T5)
      }
      event Value Change {
        n181 = event-data() -> ()  [unwired: 1 in, 2 out]
        n182 = property on="Feature List" class="MCListbox (strict)"() -> ("Value"=w343:i32)  [unwired: 2 in, 2 out]
        n183 = Index Array(array=w354, index=w343) -> (element=w360:T22)
        n184 = property on="Program step" class="LstBox (strict)"() -> ("Value"=w342:i32)  [unwired: 2 in, 2 out]
        n185 = Unbundle By Name(w360) -> ("Item Name"=w358:string, "Item Status"=w357:bool, "Steps"=w356:T23)
        n186 = Equal?(x=w342, y=-1) -> (x = y?=w346:bool)
        n187 = Select(t=0 ("y"), s=w346, f=w342) -> (s? t:f=w344:i32)
        n188 = Delete From Array(array=w356, length=1, index=w344) -> (array with subset deleted=w352:T23)  [unwired: 1 out]
        n189 = Bundle("Item Name"=w358, "Item Status"=w357, "Steps"=w352) -> (w355:T22)  [unwired: 1 in]
        n190 = call "BuildStepListFromSteps.vi"("Steps"=w352, "Control Channels"=w350, "Feedback Channels"=w349) -> ("Step List"=w348:string[])  [unwired: 12 in]
        n191 = Replace Array Subset(array=w354, new element=w355, index=w343) -> (w353:T5)
        n192 = property on="Program step" class="LstBox (strict)"("Item Names"=w348, "Value"=w344, "Key Focus"=TRUE) -> ()  [unwired: 2 in, 2 out]
      }
      event Value Change {
        n193 = event-data() -> ()  [unwired: 1 in, 1 out]
        n194 = for {
          tunnel: w363 -> [w410] mode=indexing
          tunnel: [w405] -> w371 mode=indexing
          shift-right: [w404] -> w372
          shift-left: w379 -> [w407]
          n195 = Unbundle By Name(w410) -> ("Steps"=w411:T23, "Item Name"=w409:string, "Item Status"=w408:bool)
          n196 = Array Size(array=w411) -> (size(s)=w406:i32)
          n197 = case shown="Default" w406 {
            tunnel: w411 -> [_ w418]
            tunnel: w409 -> [_ w420]
            tunnel: w408 -> [_ w419]
            tunnel: [w413 w416] -> w404
            tunnel: w407 -> [w413 w414]
            tunnel: [FALSE TRUE] -> w405
            frame 0 {
            }
            frame Default {
              n198 = Bundle("Item Name"=w420, "Item Status"=w419, "Steps"=w418) -> (w415:T22)  [unwired: 1 in]
              n199 = Build Array (concatenate)(w414, w415) -> (w416:T5)
            }
          }
        }
        n200 = And Array Elements(Boolean array=w371) -> (logical AND=w370:bool)
        n201 = case shown="True" w370 {
          tunnel: [w383 w385] -> w365
          tunnel: w364 -> [_ w393]
          tunnel: [_ w391] -> w373
          tunnel: w372 -> [_ w386]
          tunnel: enum16{"Read", "Write"}."Write" ("Read/Write") -> [_ w392]
          tunnel: "Feature List successfully saved." -> [_ w390]
          tunnel: "Error in saving Feature List." -> [_ w389]
          tunnel: "Can't save Feature List as at least one feature doesn't have steps.\nPlease check." ("message") -> [w384 w388]
          tunnel: w363 -> [w383 _]
          frame False {
            n202 = One Button Dialog(message=w384) -> ()  [unwired: 1 in, 1 out]
          }
          frame True {
            n203 = call "FileIO-ReadWrite-FeatureList.vi"("Filepath"=w393, "Feature List (In)"=w386, "Read/Write"=w392) -> ("Feature List (Out)"=w385:T5, "Error Out"=w391:errorcluster)  [unwired: 11 in]
            n204 = case shown="Error" w391 {
              tunnel: w390 -> [w394 _]
              tunnel: w389 -> [_ w395]
              tunnel: w388 -> [_ _]
              tunnel: [w394 w395] -> w387
              frame No Error {
              }
              frame Error {
              }
            }
            n205 = One Button Dialog(message=w387) -> ()  [unwired: 1 in, 1 out]
          }
        }
        n206 = disable-structure shown="Enabled" {
          frame Disabled {
            n207 = call "Program seq path.vi"() -> ()  [unwired: 11 in, 1 out]
          }
          frame Enabled {
          }
        }
        n208 = Index Array(array=w365, index=0) -> (element=w377:T22)
        n209 = Unbundle By Name(w377) -> ("Steps"=w376:T23)
        n210 = for {
          tunnel: [w402] -> w362 mode=indexing
          tunnel: w365 -> [w397] mode=indexing
          tunnel: [w396] -> _
          i -> [w396]
          n211 = Unbundle By Name(w397) -> ("Item Name"=w403:string, "Item Status"=w401:bool)
          n212 = Select(t="Active", s=w401, f="Inactive") -> (s? t:f=w398:string)
          n213 = Build Array(w403, w398) -> (w402:string[])
        }
        n214 = call "BuildStepListFromSteps.vi"("Steps"=w376, "Control Channels"=w382, "Feedback Channels"=w381, "AI"=w374) -> ("Step List"=w380:string[])  [unwired: 11 in]
        n215 = property on="Program step" class="LstBox (strict)"("Item Names"=w380, "Value"=0 ("Step feautre list")) -> ()  [unwired: 2 in, 2 out]
        n216 = property on="Feature List" class="MCListbox (strict)"("ItemNames"=w362, "Value"=0 ("Feautre list")) -> ()  [unwired: 2 in, 2 out]
      }
      event Value Change {
        n217 = event-data() -> ()  [unwired: 1 in, 1 out]
      }
      event "Program step": Double Click {
        n218 = event-data() -> ("Row"=w437:i32)  [unwired: 1 in, 8 out]
        n219 = property on="Program step" class="LstBox (strict)"() -> ("Item Names"=w438:string[])  [unwired: 2 in, 2 out]
        n220 = Index Array(array=w438, index=w437) -> (element=w428:string)
        n221 = String Length(string=w428) -> (length=w427:i32)
        n222 = String Subset(string=w428, length (rest)=2 ("length (rest)")) -> (substring=w433:string)  [unwired: 1 in]
        n223 = String Subset(string=w428, length (rest)=4 ("length (rest)")) -> (substring=w431:string)  [unwired: 1 in]
        n224 = Less Or Equal?(x=w427, y=0) -> (x <= y?=w424:bool)
        "x <= y?" <- w424
        n225 = Equal?(x=w431, y="Wait") -> (x = y?=w429:bool)
        n226 = Equal?(x=w433, y="Ch") -> (x = y?=w434:bool)
        n227 = case shown="False" w424 {
          tunnel: w446 -> [w457 _]
          tunnel: w445 -> [w456 w520]
          tunnel: w444 -> [w455 _]
          tunnel: w443 -> [w454 _]
          tunnel: w442 -> [w453 _]
          tunnel: [w452 w520] -> w441
          tunnel: [w451 w521] -> w440
          tunnel: w439 -> [w450 w521]
          tunnel: w434 -> [w449 _]
          tunnel: w429 -> [w448 _]
          tunnel: enum32{"Output", "Input"}."Output" ("y") -> [w447 _]
          frame False {
            n228 = case shown="False" w448 {
              tunnel: w457 -> [w474 w507]
              tunnel: w456 -> [w473 w506]
              tunnel: w455 -> [w472 w510]
              tunnel: w454 -> [w471 w509]
              tunnel: w453 -> [w470 w508]
              tunnel: [w469 w505] -> w452
              tunnel: [w468 w504] -> w451
              tunnel: w450 -> [w461 _]
              tunnel: w449 -> [w460 _]
              tunnel: w447 -> [w458 _]
              frame False {
                n229 = call "DO Control.vi"("s"=w460) -> ("Feedback"=w464:i32[], "Parameter (Out)"=w465:u8, "Control Channel 2"=w467:i32[], "Poll Time (Out)"=w466:u32, "Value"=w463:enum32{"Output", "Input"}, "Cancel"=w459:bool)  [unwired: 5 in]
                n230 = Equal?(x=w463, y=w458) -> (x = y?=w462:bool)
                n231 = case shown="True" w459 {
                  tunnel: w474 -> [w499 _]
                  tunnel: w473 -> [w498 w501]
                  tunnel: w472 -> [w497 _]
                  tunnel: w471 -> [w496 _]
                  tunnel: w470 -> [w495 _]
                  tunnel: [w494 w501] -> w469
                  tunnel: [w493 w502] -> w468
                  tunnel: w467 -> [w484 _]
                  tunnel: w466 -> [w483 _]
                  tunnel: w465 -> [w482 _]
                  tunnel: w464 -> [w481 _]
                  tunnel: w462 -> [w475 _]
                  tunnel: w461 -> [_ w502]
                  frame False {
                    n232 = property on="Feature List" class="MCListbox (strict)"() -> ("Value"=w485:i32)  [unwired: 2 in, 2 out]
                    n233 = Index Array(array=w498, index=w485) -> (element=w490:T22)
                    n234 = Select(t="C", s=w475, f="F") -> (s? t:f=w478:string)
                    n235 = Select(t=w484, s=w475, f=w481) -> (s? t:f=w477:i32[])
                    n236 = disable-structure shown="Disabled" {
                      disable-tunnel: w475 -> [w500 _]
                      frame Disabled {
                        n237 = call "Configuration-PromptForChannelParameters_timer.vi"("Control/Feedback\n(Default: False = Feedback)"=w500) -> ()  [unwired: 13 in, 2 out]
                      }
                      frame Enabled {
                      }
                    }
                    n238 = call "ConvertNumericChannelsToStringChannels.vi"("Channels (In)"=w477) -> ("Channels (A:B:C:D...) (Out)"=w476:string)  [unwired: 14 in]
                    n239 = Unbundle By Name(w490) -> ("Steps"=w492:T23)
                    n240 = Bundle By Name(cluster=w499, "Channel Type"=w478, "Channels"=w476, "Wait/Poll (ms)"=w483, "Parameter"=w482) -> (w491:T21)
                    n241 = property on="Program step" class="LstBox (strict)"() -> ("Value"=w486:i32)  [unwired: 2 in, 2 out]
                    n242 = Replace Array Subset(array=w492, new element=w491, index=w486) -> (w488:T23)
                    n243 = Bundle By Name(cluster=w490, "Steps"=w488) -> (w489:T22)
                    n244 = call "BuildStepListFromSteps.vi"("Steps"=w488, "Control Channels"=w495, "Feedback Channels"=w496, "AI"=w497) -> ("Step List"=w493:string[])  [unwired: 11 in]
                    "Step List 2" <- w493
                    n245 = Replace Array Subset(array=w498, new element=w489, index=w485) -> (w494:T5)
                    n246 = property on="Program step" class="LstBox (strict)"("Key Focus"=TRUE, "Value"=w486, "Item Names"=w493) -> ()  [unwired: 2 in, 2 out]
                  }
                  frame True {
                  }
                }
              }
              frame True {
                n247 = property on="Feature List" class="MCListbox (strict)"() -> ("Value"=w511:i32)  [unwired: 2 in, 2 out]
                n248 = call "Timer.vi"() -> ("Wait Time out"=w503:u32)  [unwired: 10 in, 1 out]
                n249 = Index Array(array=w506, index=w511) -> (element=w515:T22)
                n250 = Bundle By Name(cluster=w507, "Channel Type"="N", "Wait/Poll (ms)"=w503) -> (w517:T21)
                n251 = Unbundle By Name(w515) -> ("Steps"=w516:T23)
                n252 = property on="Program step" class="LstBox (strict)"() -> ("Value"=w518:i32)  [unwired: 2 in, 2 out]
                n253 = Replace Array Subset(array=w516, new element=w517, index=w518) -> (w513:T23)
                n254 = Bundle By Name(cluster=w515, "Steps"=w513) -> (w514:T22)
                n255 = call "BuildStepListFromSteps.vi"("Steps"=w513, "Control Channels"=w508, "Feedback Channels"=w509, "AI"=w510) -> ("Step List"=w504:string[])  [unwired: 11 in]
                n256 = property on="Program step" class="LstBox (strict)"("Item Names"=w504, "Value"=w518, "Key Focus"=TRUE) -> ()  [unwired: 2 in, 2 out]
                n257 = Replace Array Subset(array=w506, new element=w514, index=w511) -> (w505:T5)
              }
            }
          }
          frame True {
          }
        }
      }
      event Panel Close? {
        n258 = event-data() -> ()  [unwired: 1 in, 1 out]
        n259 = event-data("Discard?"=TRUE) -> ()  [unwired: 1 in, 1 out]
      }
    }
  }
  "Error Out" <- w24
